vi "Init Valve.vi"(7 "VolatusAPI":refnum<class "VolatusAPI.lvclass">, 8 "error in (no error)":errorcluster, 10 "Config Element":refnum<class "Config Element.lvclass">, 11 "LatchedValve in":refnum<class "LatchedValve.lvclass">) -> (0 "error out":errorcluster, 3 "LatchedValve out":refnum<class "LatchedValve.lvclass">)   [LabVIEW 2020, in "VolatusControl.lvlib" / "LatchedValve.lvclass"]
uses:
  LatchedValve.lvclass
  LatchedValve.lvclass/LatchedValve.ctl
  lv-cdm/CDM-Config/Config Element/Config Element.lvclass
  Volatus/VolatusAPI/VolatusAPI.lvclass
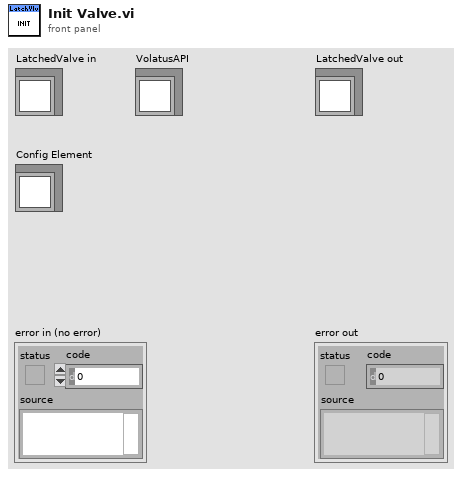
[diagram p1: front panel]
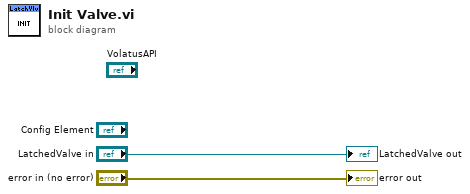
[diagram p0: block diagram]
diagram:
  "error out" <- "error in (no error)"
  "LatchedValve out" <- "LatchedValve in"
